vi "关键参数存表.vi"(8 "error in (no error)":errorcluster, 9 "仪器参数":T2 {"单位" items=["ug/L", "mg/L"]}, 10 "datatime":timestamp, 11 "仪器名称":string) -> (0 "error out":errorcluster)   [LabVIEW 2016, in "斯坦道总磷.lvlib"]
panel:
  in  "database":string="database3.mdb"
  in  "table":string="仪器参数"
  out "data in":T1={"时间标识"=timestamp(0 s since 1904-01-01), "仪器参数"="", "测量量程"=0.0, "测量精度"=0.0, "测量间隔"=0.0, "消解温度"=0.0, "消解时长"=0.0, "空白校准时间"=timestamp(0 s since 1904-01-01), "曲线截距"=0.0, "曲线斜率"=0.0, "测量检出限"=0.0, "测量信号值"=0.0, "线性相关系数"=0.0, "二次多项式系数"=0.0, "标样校准时间"=timestamp(0 s since 1904-01-01), "单位"=enum."mg/L"}
  out "columns":string[](array[string])
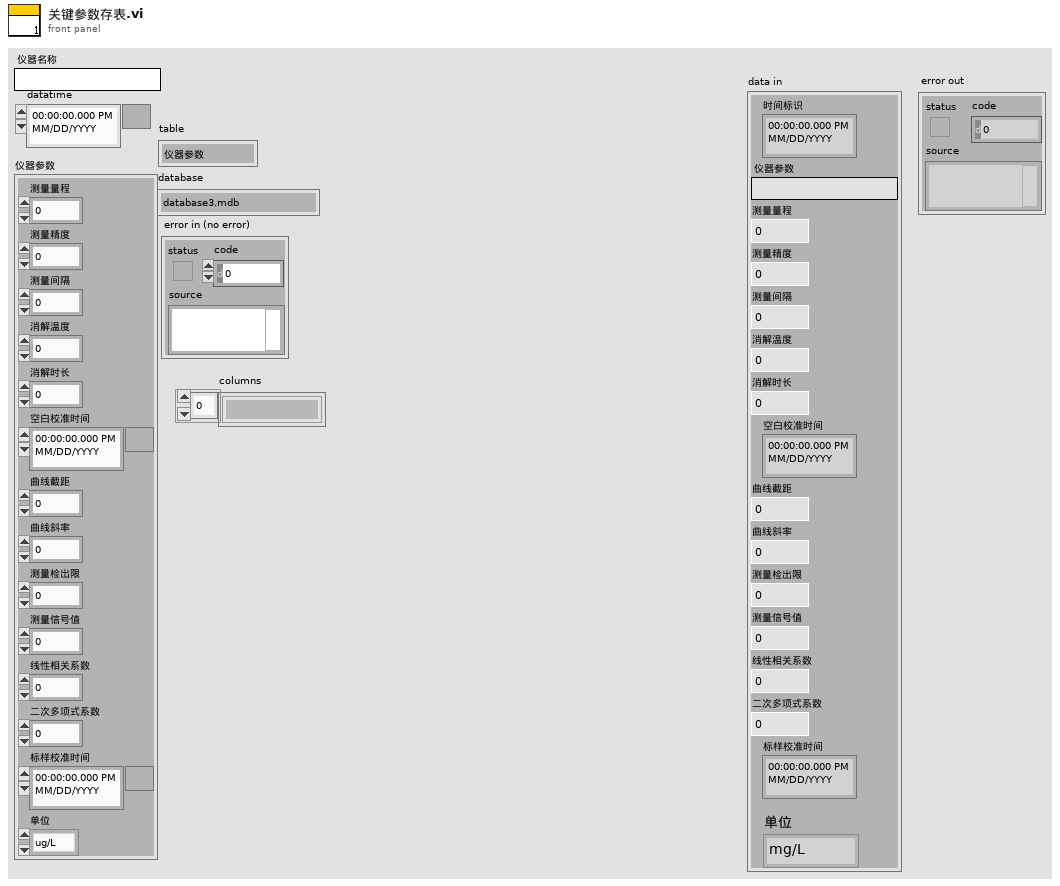
[diagram p1: front panel]
types:
  T1 = cluster{"时间标识":timestamp, "仪器参数":string, "测量量程":dbl, "测量精度":dbl, "测量间隔":dbl, "消解温度":dbl, "消解时长":dbl, "空白校准时间":timestamp, "曲线截距":dbl, "曲线斜率":dbl, "测量检出限":dbl, "测量信号值":dbl, "线性相关系数":dbl, "二次多项式系数":dbl, "标样校准时间":timestamp, "单位":enum16{"ug/L", "mg/L"}}
  T2 = cluster{"测量量程":dbl, "测量精度":dbl, "测量间隔":dbl, "消解温度":dbl, "消解时长":dbl, "空白校准时间":timestamp, "曲线截距":dbl, "曲线斜率":dbl, "测量检出限":dbl, "测量信号值":dbl, "线性相关系数":dbl, "二次多项式系数":dbl, "标样校准时间":timestamp, "单位":u16}
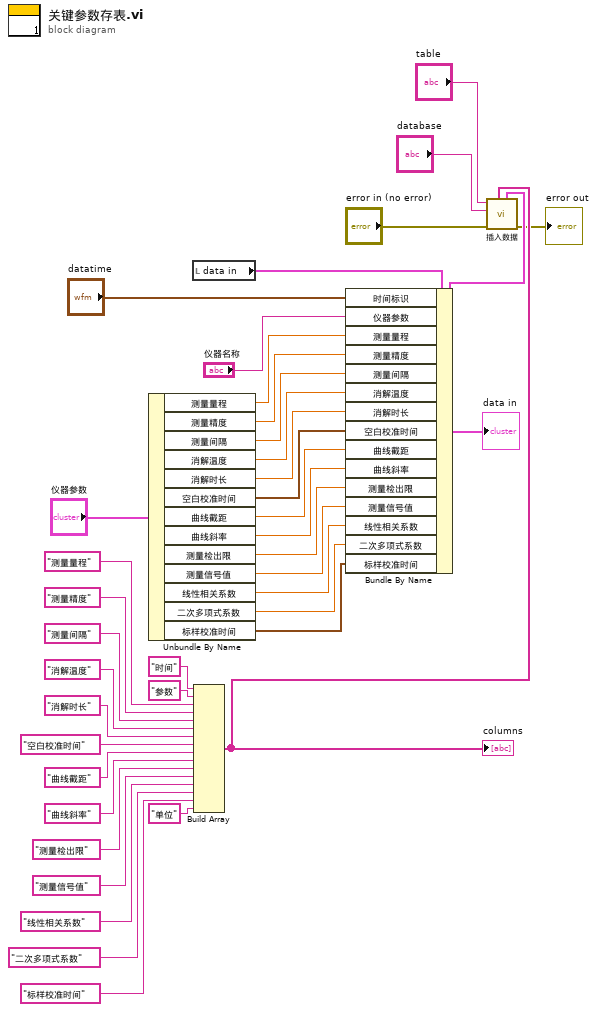
[diagram p0: block diagram]
diagram:
  n1 = Unbundle By Name("仪器参数") -> ("测量量程"=w23:dbl, "测量精度"=w22:dbl, "测量间隔"=w21:dbl, "消解温度"=w20:dbl, "消解时长"=w19:dbl, "空白校准时间"=w18:timestamp, "曲线截距"=w17:dbl, "曲线斜率"=w16:dbl, "测量检出限"=w15:dbl, "测量信号值"=w14:dbl, "线性相关系数"=w13:dbl, "二次多项式系数"=w12:dbl, "标样校准时间"=w11:timestamp)
  n2 = local read "data in"() -> (w9:T1)
  n3 = Build Array("时间" ("元素"), "参数" ("元素"), "测量量程", "测量精度" ("元素"), "测量间隔", "消解温度", "消解时长", "空白校准时间", "曲线截距", "曲线斜率", "测量检出限", "测量信号值", "线性相关系数", "二次多项式系数", "标样校准时间", "单位" ("元素")) -> (w6:string[])
  "columns" <- w6
  n4 = Bundle By Name(cluster=w9, "时间标识"="datatime", "仪器参数"="仪器名称", "测量量程"=w23, "测量精度"=w22, "测量间隔"=w21, "消解温度"=w20, "消解时长"=w19, "空白校准时间"=w18, "曲线截距"=w17, "曲线斜率"=w16, "测量检出限"=w15, "测量信号值"=w14, "线性相关系数"=w13, "二次多项式系数"=w12, "标样校准时间"=w11) -> (w5:T1)
  "data in" <- w5
  n5 = call "插入数据.vi"("data"=w5, "columns"=w6, "error in (no error)"="error in (no error)", "database"="database", "table"="table") -> ("error out"=→"error out":errorcluster)  [unwired: 6 in]
